vi "Read MFC.vi"(8 "error in (no error)":errorcluster, 11 "MFC in":refnum<class "Valve.lvclass">) -> (0 "error out":errorcluster, 3 "MFC out":refnum<class "Valve.lvclass">)   [LabVIEW 2013]
uses:
  Valve.lvclass
  Valve Messages/Update Graphs Msg/Update Graphs Msg.lvclass
  PluginInterface/Actor Framework.lvlibp/Actor/Actor.lvclass
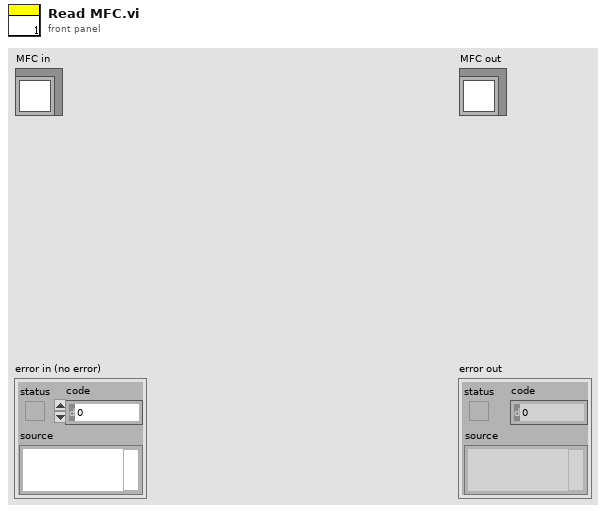
[diagram p1: front panel]
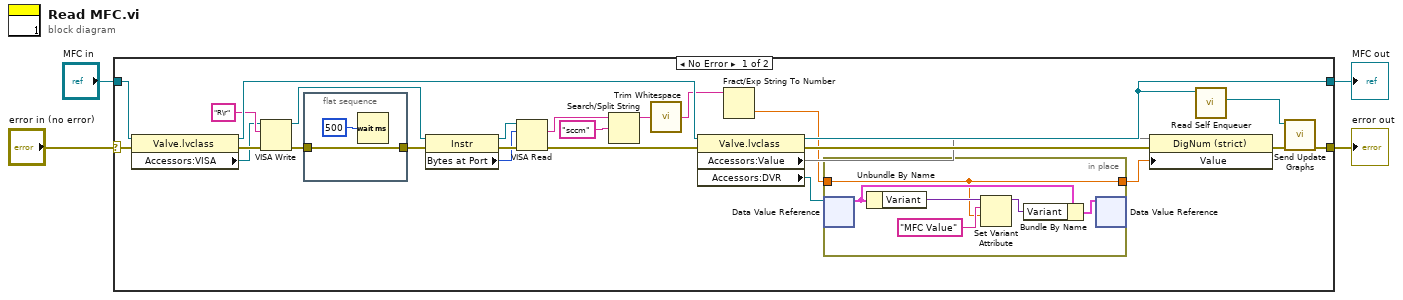
[diagram p0: block diagram]
diagram:
  n1 = case shown="No Error" "error in (no error)" {
    selector: "error in (no error)" -> [w29 w40]
    tunnel: [w22 w40] -> w3
    tunnel: [w24 w39] -> w1
    tunnel: "MFC in" -> [w30 w39]
    frame No Error {
      n2 = property class="Valve.lvclass"(reference=w30, error in=w29) -> (reference out=w26:refnum<class "Valve.lvclass">, error out=w28:errorcluster, "Accessors:VISA"=w10:refnum<visa-resource-name>)
      n3 = VISA Write(VISA resource name=w10, write buffer="R\r", error in (no error)=w28) -> (VISA resource name out=w20:refnum<visa-resource-name>, error out=w17:errorcluster)  [unwired: 1 out]
      n4 = flat-sequence {
        tunnel: [w37] -> w18
        tunnel: w17 -> [w37]
        frame #0 {
          n5 = Wait (ms)(milliseconds to wait=u32 500) -> ()  [unwired: 1 out]
        }
      }
      n6 = property class="Instr"(reference=w20, error in=w18) -> (reference out=w21:refnum<visa-resource-name>, error out=w19:errorcluster, "Bytes at Port"=w15:u32)
      n7 = VISA Read(VISA resource name=w21, byte count=w15, error in (no error)=w19) -> (read buffer=w11:string, error out=w25:errorcluster)  [unwired: 2 out]
      n8 = Search/Split String(string=w11, search string/char (-)="sccm") -> (substring before match=w13:string)  [unwired: 1 in, 2 out]
      n9 = call <vilib>:"Trim Whitespace.vi"("string"=w13) -> ("trimmed string"=w12:string)  [unwired: 1 in]
      n10 = property class="Valve.lvclass"(reference=w26, error in=w25) -> (reference out=w24:refnum<class "Valve.lvclass">, error out=w27:errorcluster, "Accessors:Value"=w7, "Accessors:DVR"=w8:refnum<data-value>)
      n11 = Fract/Exp String To Number(string=w12) -> (number=w6:dbl)  [unwired: 3 in, 1 out]
      n12 = in-place {
        in-place-border: w6 -> [w31]
        in-place-border: [w31] -> w5
        n13 = in-place-dvr #1(w8) -> (w33:cluster{"Array":string[], "Variant":variant})  [unwired: 1 out]
        n14 = Unbundle By Name(w33) -> ("Variant"=w35:variant)
        n15 = Set Variant Attribute(Variant=w35, name="MFC Value", value=w31) -> (Variant out=w34:variant)  [unwired: 1 in, 2 out]
        n16 = Bundle By Name(cluster=w33, "Variant"=w34) -> (w36:cluster{"Array":string[], "Variant":variant})
        n17 = in-place-dvr #1(w36) -> ()  [unwired: 2 out]
      }
      n18 = property class="DigNum (strict)"(reference=w7, error in=w27, "Value"=w5) -> (error out=w9:errorcluster)  [unwired: 1 out]
      n19 = call "Read Self Enqueuer.vi"("Actor"=w24) -> ("Self Enqueuer"=w23:refnum<class "Message Enqueuer.lvclass">)  [unwired: 10 in]
      n20 = call "Send Update Graphs.vi"("error in (no error)"=w9, "Message Enqueuer"=w23) -> ("error out"=w22:errorcluster)  [unwired: 8 in, 1 out]
    }
    frame Error {
    }
  }
  "error out" <- w3
  "MFC out" <- w1
